vi "Write Close.vi"(0 "EnclaveChannel":T1) -> ()   [LabVIEW 2022 SP3, in "Enclave.lvlib"]
uses:
  Enclave.lvlib
  ))Channel.ctl
  Element.ctl
  Operation.ctl
  Enclave/Enclave.lvclass
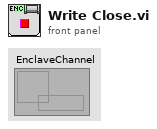
[diagram p1: front panel]
types:
  T1 = typedef "Enclave.lvlib/))Channel.ctl" = refnum<queue>
  T2 = typedef "Enclave.lvlib/Operation.ctl" = enum16{"Get Core", "Init", "Close"}
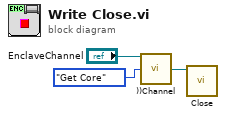
[diagram p0: block diagram]
diagram:
  n1 = call "))Channel.vi"("EnclaveChannel in"="EnclaveChannel", "Operation"=Operation."Get Core") -> ("Enclave"=w1:refnum<class "Enclave.lvclass">)  [unwired: 11 in, 2 out]
  n2 = call "Close.vi"("Enclave in"=w1) -> ()  [unwired: 10 in, 1 out]
